vi "流量计全局变量.vi"() -> ()   [LabVIEW 2016, in "流量计集成.lvlib"]
panel:
  in  "运行模式设置":enum16{"按周期模式", "全常规模式"}(ring)=enum."全常规模式"
  in  "运行模式":enum16{"维护模式", "常规模式", "应急模式", "质控模式"}(ring)=enum."常规模式"
  in  "数量 5":u16
  in  "流量计启用 5":bool
  in  "流量计类型":T1
  in  "数量 4":u16
  in  "流量计启用 4":bool
  in  "流量计启用 3":bool
  in  "流量计启用 2":bool
  in  "流量计启用":bool
  in  "博意达流量计启用":bool[](array[boolean])
  in  "运行间隔":i16=4 min=1 max=24
  in  "数量 3":u16
  in  "数量 2":u16
  in  "数量":u16
  out "总累积流量":dbl
  out "总流量":dbl
  out "平均流速":dbl
  out "平均水位":dbl
  out "TX Timestamp":timestamp
  out "TX Data":string
  out "RX Timestamp":timestamp
  out "RX Data":string
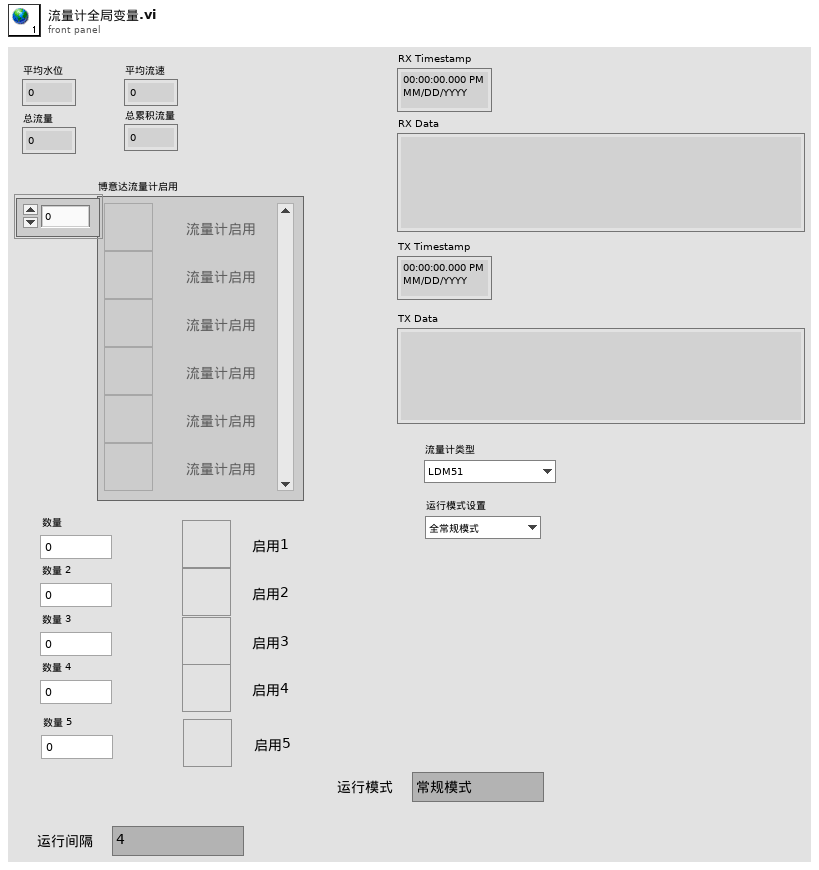
[diagram p1: front panel]
types:
  T1 = typedef "流量计集成.lvlib/流量计类型.ctl" = enum16{"LDM51", "MGG/KL QC", "斯坦道功率测流", "博意达流量计", "SL1500-3G", "WL1A1明渠流量计"}
diagram:
